vi "FPGA Simulation.vi"() -> ()   [LabVIEW 2014]
uses:
  <vilib>/rvi/DesktopExecutionNode/DesktopExecutionNode.xnode
  <vilib>/rvi/DesktopExecutionNode/Execution/niFpgaDEN_Execute.vi
panel:
  in  "stop":bool
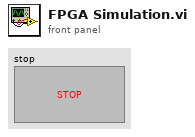
[diagram p1: front panel]
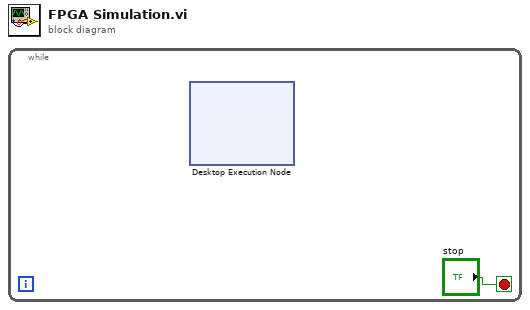
[diagram p0: block diagram]
diagram:
  n1 = while {
    stop <- "stop" stop-if-true
    n2 = xnode "Desktop Execution Node"() -> ()  [unwired: 1 in, 1 out]
  }
